vi "ExtractTrigger.vi"(3 "All Info":T1 {"Data Set"."Settings"."Time" format="%<%H:%M\n%d/%m/%y>T"; "task ID" format="%.0x"}, 4 "Trigger":dbl, 5 "All Info":T1 {"Data Set"."Settings"."Time" format="%<%H:%M\n%d/%m/%y>T"; "task ID" format="%.0x"}) -> (0 "Data Set":T2[](array[typedef]) {"Settings"."Time" format="%<%H:%M\n%d/%m/%y>T"}, 1 "Trigger?":bool, 2 "All Info":T1 {"Data Set"."Settings"."Time" format="%<%H:%M\n%d/%m/%y>T"; "task ID" format="%.0x"})   [LabVIEW 2014]
uses:
  <userlib>/CurtinCode/AllDataCtrl.ctl
  <userlib>/CurtinCode/DataControl.ctl
  <userlib>/CurtinCode/SettingsControl.ctl
  <vilib>/sound2/lvsound2.llb/Sound Input Task ID.ctl
panel:
  out "Waveform Graph":dbl[][](graph)
  in  "Tab Control":enum32{"Last Run", "Last Last Run", "Out"}(tab)
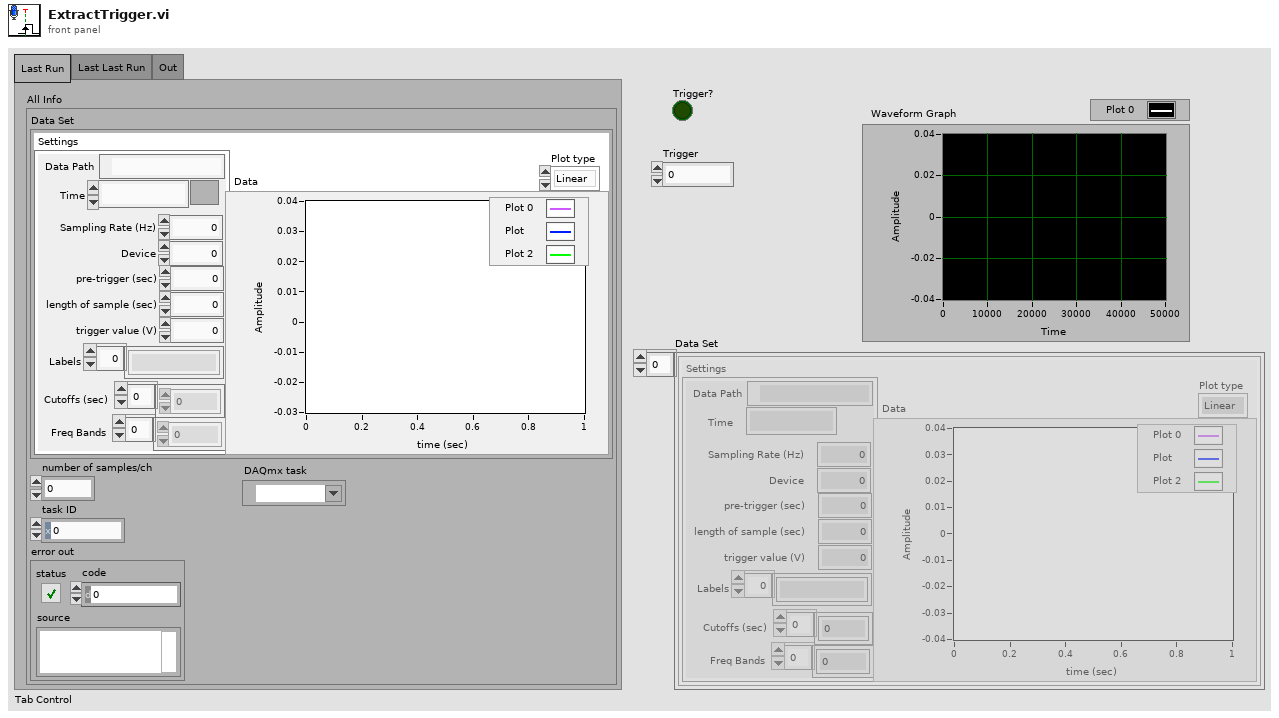
[diagram p1: front panel]
types:
  T1 = typedef "AllDataCtrl.ctl" = cluster{"Data Set":T2, "number of samples/ch":i32, "task ID":T4, "error out":errorcluster, "DAQmx task":refnum<k21>}
  T2 = typedef "DataControl.ctl" = cluster{"Settings":T3, "Data":cluster{i32, dbl, "data":dbl[]}[], "Plot type":enum16{"Linear", "log"}}
  T3 = typedef "SettingsControl.ctl" = cluster{"Data Path":path, "Time":timestamp, "Sampling Rate (Hz)":u16, "Device":u16, "pre-trigger (sec)":dbl, "length of sample (sec)":dbl, "trigger value (V)":dbl, "Labels":string[], "Cutoffs (sec)":dbl[], "Freq Bands":dbl[]}
  T4 = typedef "Sound Input Task ID.ctl" = u32
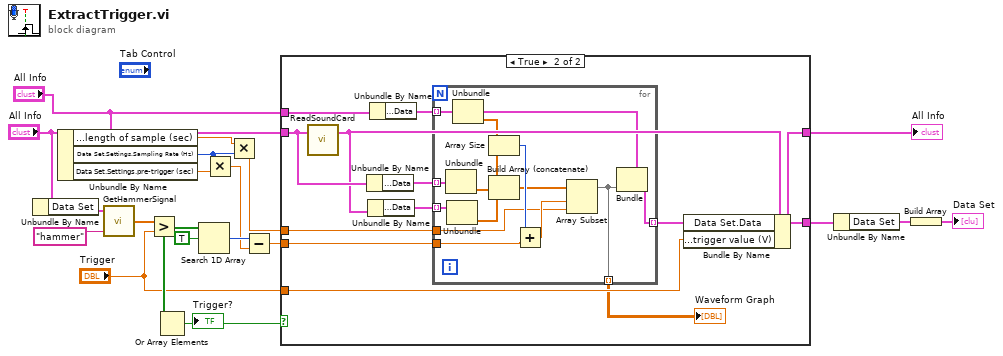
[diagram p0: block diagram]
diagram:
  n1 = Unbundle By Name("All Info") -> ("Data Set"=w18:T2)
  n2 = Unbundle By Name("All Info") -> ("Data Set.Settings.length of sample (sec)"=w6:dbl, "Data Set.Settings.Sampling Rate (Hz)"=w7:u16, "Data Set.Settings.pre-trigger (sec)"=w11:dbl)
  n3 = call <userlib>:"GetHammerSignal.vi"("column"="hammer", "Data Set"=w18) -> ("Data set"=w1:dbl[])  [unwired: 1 in, 2 out]
  n4 = Greater?(x=w1, y="Trigger") -> (0:w14:bool[])
  n5 = Or Array Elements(Boolean array=w14) -> (logical OR=w19:bool)
  "Trigger?" <- w19
  n6 = Search 1D Array(1D array=w14, element=TRUE) -> (index of element=w10:i32)  [unwired: 1 in]
  n7 = Multiply(x=w7, y=w11) -> (x*y=w9:dbl)
  n8 = Multiply(x=w6, y=w7) -> (x*y=w5:dbl)
  n9 = Subtract(x=w10, y=w9) -> (x-y=w8:dbl)
  n10 = case shown="True" w19 {
    tunnel: "All Info" -> [_ w33]
    tunnel: "All Info" -> [w21 w32]
    tunnel: [w21 w24] -> w3
    tunnel: [_ w24] -> w4
    tunnel: w8 -> [_ w26]
    tunnel: w5 -> [_ w25]
    tunnel: "Trigger" -> [_ w23]
    frame False {
    }
    frame True {
      n11 = call <userlib>:"ReadSoundCard.vi"("All Info"=w32) -> ("All Info"=w28:T1)  [unwired: 1 in, 1 out]
      n12 = Unbundle By Name(w32) -> ("Data Set.Data"=w29:cluster{i32, dbl, "data":dbl[]}[])
      n13 = Unbundle By Name(w28) -> ("Data Set.Data"=w30:cluster{i32, dbl, "data":dbl[]}[])
      n14 = Unbundle By Name(w33) -> ("Data Set.Data"=w31:cluster{i32, dbl, "data":dbl[]}[])
      n15 = for {
        tunnel: w31 -> [w42] mode=indexing
        tunnel: w30 -> [w46] mode=indexing
        tunnel: w29 -> [w45] mode=indexing
        tunnel: [w41] -> w27 mode=indexing
        tunnel: w26 -> [w38]
        tunnel: w25 -> [w35]
        tunnel: [w34] -> w22 mode=indexing
        n16 = Unbundle(w45) -> ("data"=w44:dbl[])  [unwired: 2 out]
        n17 = Unbundle(w46) -> ("data"=w43:dbl[])  [unwired: 2 out]
        n18 = Unbundle(w42) -> ("data"=w40:dbl[])  [unwired: 2 out]
        n19 = Array Size(array=w40) -> (size(s)=w39:i32)
        n20 = Build Array (concatenate)(w40, w44, w43) -> (w37:dbl[])
        n21 = Add(x=w39, y=w38) -> (x+y=w36:dbl)
        n22 = Array Subset(array=w37, index=w36, length=w35) -> (w34:dbl[])
        n23 = Bundle(cluster=w42, "data"=w34) -> (w41:cluster{i32, dbl, "data":dbl[]})  [unwired: 2 in]
      }
      "Waveform Graph" <- w22
      n24 = Bundle By Name(cluster=w28, "Data Set.Data"=w27, "Data Set.Settings.trigger value (V)"=w23) -> (w24:T1)
    }
  }
  "All Info" <- w3
  n25 = Unbundle By Name(w4) -> ("Data Set"=w15:T2)
  n26 = Build Array(w15) -> (→"Data Set":T2[])
